vi "Save_Source_Type.vi"(8 "error in (no error)":errorcluster, 9 "index in":string, 10 "buildObject":T1, 11 "Class in":refnum<class "IB_CGen.lvclass">) -> (0 "error out":errorcluster, 1 "index out":string, 2 "buildObject out":T1, 3 "Class out":refnum<class "IB_CGen.lvclass">)   [LabVIEW 2020, in "IB_CGen.lvclass"]
uses:
  <vilib>/AppBuilder/IB_Classes/Source/Container/Build/CGen/IB_CGen.lvclass
  <vilib>/AppBuilder/IB_Classes/Source/Container/Build/CGen/IB_CGen.lvclass/IB_CGen.ctl
  <resource>/Framework/Providers/API/ItemRef.ctl
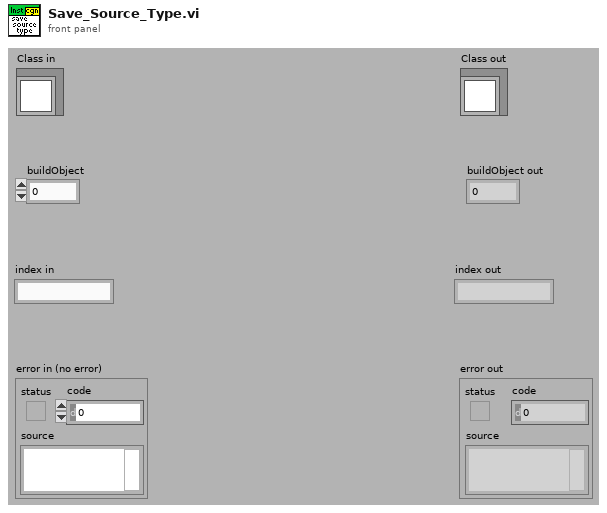
[diagram p1: front panel]
types:
  T1 = typedef "ItemRef.ctl" = u64
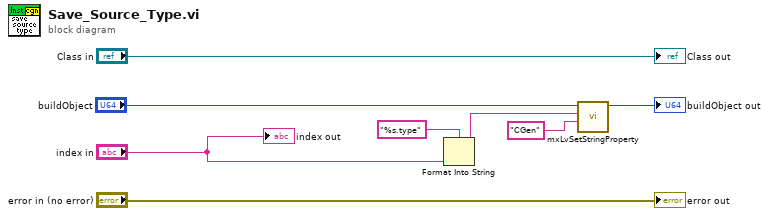
[diagram p0: block diagram]
diagram:
  n1 = Format Into String(format string="%s.type", "index in") -> (resulting string=w7:string)  [unwired: 2 in, 1 out]
  n2 = call <resource>:"mxLvSetStringProperty.vi"("Value (\"\")"="CGen" ("Value (\"\")"), "Tag"=w7, "Item"="buildObject") -> ("Item"=→"buildObject out":T1)  [unwired: 2 in, 6 out]
  "error out" <- "error in (no error)"
  "Class out" <- "Class in"
  "index out" <- "index in"
